vi "registerPublishers.vi"(8 "error in (no error)":errorcluster, 11 "MonoPubSubData in":refnum<class "MonoPubSubData.lvclass">) -> (0 "error out":errorcluster, 2 "publishersRegs":refnum<event-registration>, 3 "MonoPubSubData out":refnum<class "MonoPubSubData.lvclass">)   [LabVIEW 2020, in "MonoPubSubData.lvclass"]
uses:
  MonoPubSubData.lvclass
  Typedefs/wavelength.ctl
  Typedefs/DeviceStatus.ctl
  Typedefs/GratingType.ctl
  Typedefs/slit.ctl
  Typedefs/SlitType.ctl
  Typedefs/slitWidth.ctl
  MonoPubSubData.lvclass/MonoPubSubData.ctl
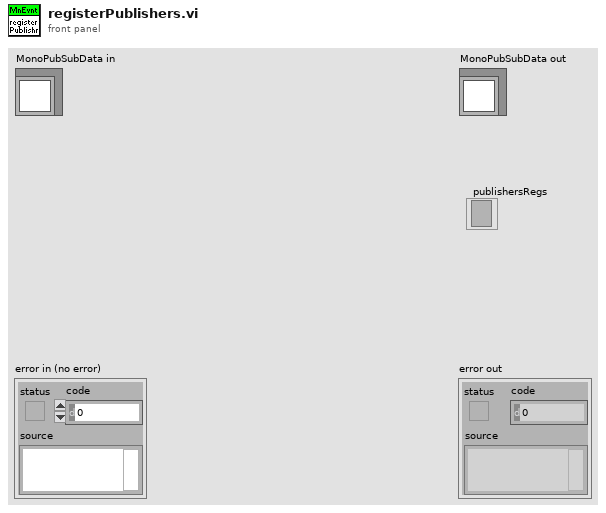
[diagram p1: front panel]
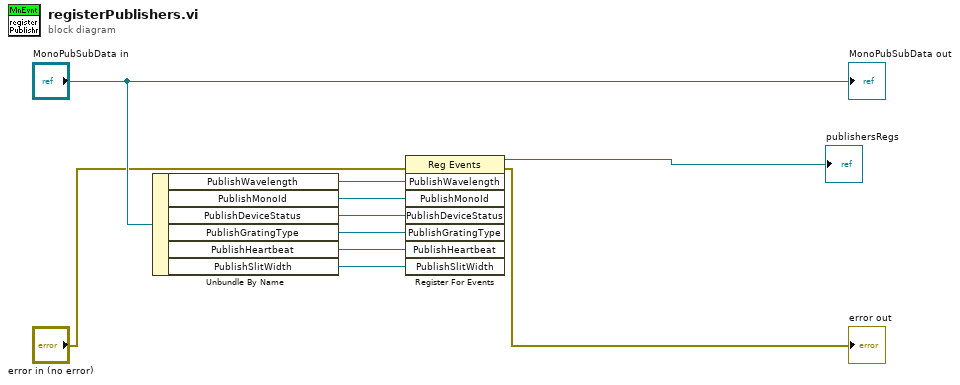
[diagram p0: block diagram]
diagram:
  n1 = Unbundle By Name("MonoPubSubData in") -> ("PublishWavelength"=w9:refnum<user-event>, "PublishMonoId"=w8:refnum<user-event>, "PublishDeviceStatus"=w7:refnum<user-event>, "PublishGratingType"=w6:refnum<user-event>, "PublishHeartbeat"=w5:refnum<user-event>, "PublishSlitWidth"=w4:refnum<user-event>)
  n2 = register-events(error in="error in (no error)", w9, w8, w7, w6, w5, w4) -> (reference out=→"publishersRegs":refnum<event-registration>, error out=→"error out":errorcluster)  [unwired: 1 in]
  "MonoPubSubData out" <- "MonoPubSubData in"
